vi "Get Build Log.vi"(0 "Export In":refnum<class "Export.lvclass">, 11 "error in (no error)":errorcluster) -> (4 "Export Out":refnum<class "Export.lvclass">, 6 "Log":string, 15 "error out":errorcluster)   [LabVIEW 2017, in "CL_G3_VIComponentBuilder.lvlib" / "Export.lvclass"]
doc: "Returns the log of operations during the export artifacts' creation."
uses:
  Export.lvclass
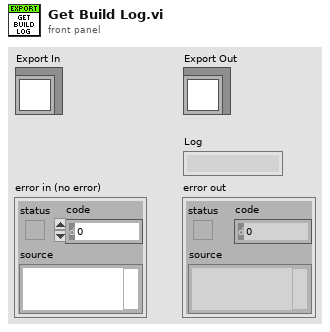
[diagram p1: front panel]
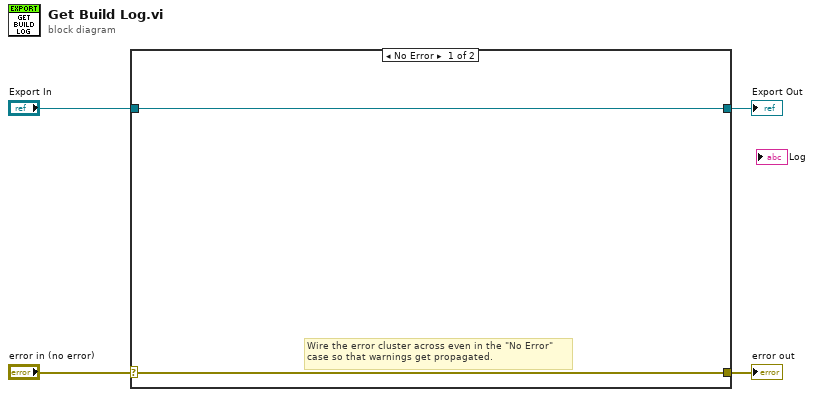
[diagram p0: block diagram]
diagram:
  n1 = case shown="No Error" "error in (no error)" {
    selector: "error in (no error)" -> [w5 w8]
    tunnel: [w5 w8] -> w3
    tunnel: [w6 w7] -> w1
    tunnel: "Export In" -> [w6 w7]
    frame No Error {
      # "Wire the error cluster across even in the \"No Error\"\ncase so that warnings get propagated."
    }
    frame Error {
    }
  }
  "error out" <- w3
  "Export Out" <- w1
